vi "Set Initial Value.vi"(8 "error in (no error)":errorcluster, 10 "Default Value":variant, 11 "Control in":refnum<class "Control.lvclass">) -> (0 "error out":errorcluster, 3 "Control out":refnum<class "Control.lvclass">)   [LabVIEW 2020, in "Aether Engine.lvlib" / "Control.lvclass"]
uses:
  Control.lvclass
  Control.lvclass/Control.ctl
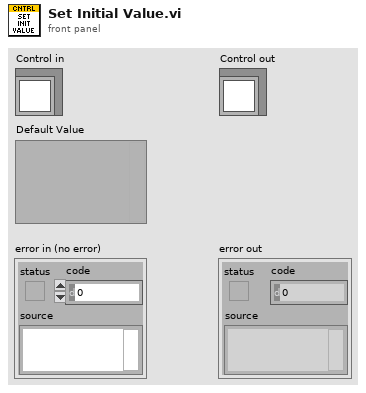
[diagram p1: front panel]
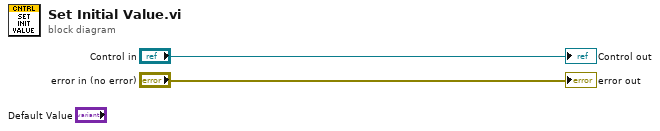
[diagram p0: block diagram]
diagram:
  "error out" <- "error in (no error)"
  "Control out" <- "Control in"
